vi "updateNode.vi"(0 "ROS_Master in":refnum<class "ROS_Master.lvclass">, 1 "PubSub in":T1) -> (2 "ROS_Master out":refnum<class "ROS_Master.lvclass">, 3 "Shutdown URI":string, 4 "shutdown needed?":bool)   [LabVIEW 2012, in "ROS_Master.lvclass"]
uses:
  <userlib>/ROSforLV/ROS/Code/ROS_Master/ROS_Master.lvclass
  <userlib>/ROSforLV/ROS/Code/ROS_Master/ROS_Master.lvclass/ROS_Master.ctl
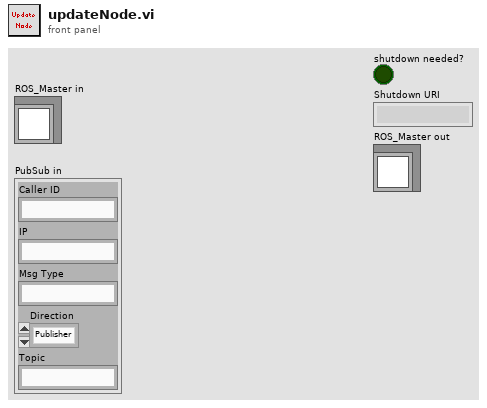
[diagram p1: front panel]
types:
  T1 = cluster{"Caller ID":string, "IP":string, "Msg Type":string, "Direction":enum16{"Publisher", "Subscriber"}, "Topic":string}
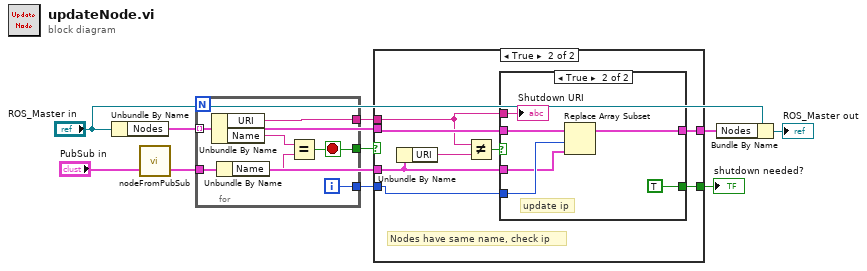
[diagram p0: block diagram]
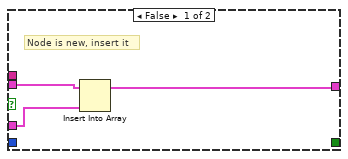
[diagram p2: hidden frame]
diagram:
  n1 = Unbundle By Name("ROS_Master in") -> ("Nodes"=w8:cluster{"Name":string, "URI":string}[])
  n2 = call <userlib>:"nodeFromPubSub.vi"("PubSub in"="PubSub in") -> ("Node"=w4:cluster{"Name":string, "URI":string})  [unwired: 2 in]
  n3 = for {
    tunnel: w4 -> [w16]
    tunnel: w8 -> [w17] mode=indexing
    tunnel: [w13] -> w10
    tunnel: [w12] -> w9
    tunnel: [w11] -> w7
    i -> [w11]
    stop <- w13 stop-if-true
    n4 = Unbundle By Name(w17) -> ("URI"=w12:string, "Name"=w15:string)
    n5 = Unbundle By Name(w16) -> ("Name"=w14:string)
    n6 = Equal?(x=w15, y=w14) -> (x = y?=w13:bool)
  }
  n7 = case shown="True" w10 {
    tunnel: w9 -> [_ w21]
    tunnel: w4 -> [w19 w24]
    tunnel: w8 -> [w20 w26]
    tunnel: w7 -> [_ w25]
    tunnel: [_ w27] -> w6
    tunnel: [w18 w22] -> w2
    frame False {
      # "Node is new, insert it"
      n8 = Insert Into Array(array=w20, new element=w19) -> (w18:cluster{"Name":string, "URI":string}[])  [unwired: 1 in]
    }
    frame True {
      # "Nodes have same name, check ip"
      n9 = Unbundle By Name(w24) -> ("URI"=w23:string)
      n10 = Not Equal?(x=w21, y=w23) -> (x != y?=w28:bool)
      n11 = case shown="True" w28 {
        tunnel: [_ TRUE] -> w27
        tunnel: w26 -> [w29 w34]
        tunnel: w25 -> [_ w33]
        tunnel: w24 -> [_ w32]
        tunnel: [w29 w31] -> w22
        tunnel: w21 -> [_ w30]
        frame False {
        }
        frame True {
          # "update ip"
          n12 = Replace Array Subset(array=w34, new element=w32, index=w33) -> (w31:cluster{"Name":string, "URI":string}[])
          "Shutdown URI" <- w30
        }
      }
    }
  }
  "shutdown needed?" <- w6
  n13 = Bundle By Name(cluster="ROS_Master in", "Nodes"=w2) -> (→"ROS_Master out":refnum<class "ROS_Master.lvclass">)
